vi "Errors Registered.vi"(8 "error in (no error)":errorcluster, 9 "Operation":T5, 11 "Error Info":T1 {"Context"."name" items=["Method Name", "Parameter Name", "VI Name", "Control Name", "Proxy Dll Path", "Project Library Name"]; "Error Number" items=["ERR_NOERROR"=0, "ERR_ACCESS_OUTPUTFOLDER"=1, "ERR_INVALID_LIBRARYNAME"=2, "ERR_CREATE_VIWRAPPER"=3, "ERR_UNKNOWN"=201, "ERR_BAD_ARGUMENT"=202, "ERR_URL_NOTFOUND_BADWSDL"=203, "ERR_BADLYFORMATTEDURL"=204, "ERR_BADHOSTNAME"=205, "ERR_BADDIRECTORY"=206, "ERR_UNAUTHORIZEDACCESS"=207, "ERR_CREATELIBRARY"=208, "ERR_COMPILEERROR"=209]}) -> (0 "error out":errorcluster, 3 "Array (out)":T1[](array[typedef]) {"Context"."name" items=["Method Name", "Parameter Name", "VI Name", "Control Name", "Proxy Dll Path", "Project Library Name"]; "Error Number" items=["ERR_NOERROR"=0, "ERR_ACCESS_OUTPUTFOLDER"=1, "ERR_INVALID_LIBRARYNAME"=2, "ERR_CREATE_VIWRAPPER"=3, "ERR_UNKNOWN"=201, "ERR_BAD_ARGUMENT"=202, "ERR_URL_NOTFOUND_BADWSDL"=203, "ERR_BADLYFORMATTEDURL"=204, "ERR_BADHOSTNAME"=205, "ERR_BADDIRECTORY"=206, "ERR_UNAUTHORIZEDACCESS"=207, "ERR_CREATELIBRARY"=208, "ERR_COMPILEERROR"=209]})   [LabVIEW 2020, in "WebServiceImporter.lvlib" / "Error Handling.lvlib"]
uses:
  <vilib>/Platform/WebService/Error Handling/Error Handling.lvlib
  <vilib>/Platform/WebService/Error Handling/Error/Operation.ctl
  <vilib>/Platform/WebService/Error Handling/Error/Error Info.ctl
  <vilib>/Platform/WebService/Error Handling/Error/Error Number.ctl
  <vilib>/Platform/WebService/Error Handling/Error/Context.ctl
  <vilib>/Platform/WebService/Error Handling/Error/Context Name.ctl
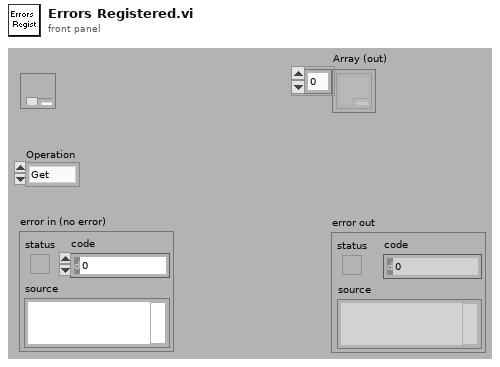
[diagram p1: front panel]
types:
  T1 = typedef "WebServiceImporter.lvlib/Error Handling.lvlib/Error Info.ctl" = cluster{"Specifics":string, "Error Number":T2, "Call Chain":string, "Context":T3}
  T2 = typedef "WebServiceImporter.lvlib/Error Handling.lvlib/Error Number.ctl" = u16
  T3 = typedef "WebServiceImporter.lvlib/Error Handling.lvlib/Context.ctl" = cluster{"name":T4, "value":string}[]
  T4 = typedef "WebServiceImporter.lvlib/Error Handling.lvlib/Context Name.ctl" = u16
  T5 = typedef "WebServiceImporter.lvlib/Error Handling.lvlib/Operation.ctl" = enum16{"Get", "Add", "Clear"}
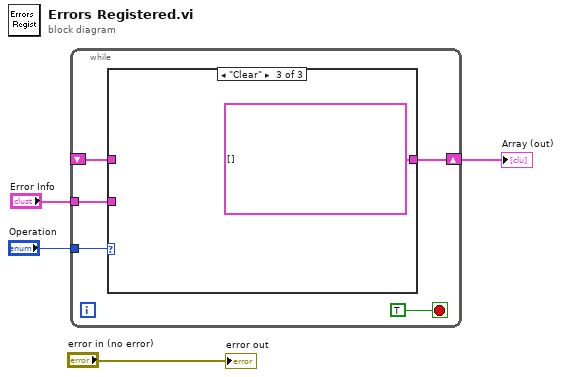
[diagram p0: block diagram]
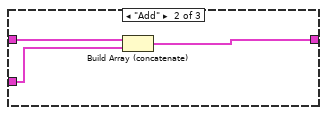
[diagram p3: hidden frame]
diagram:
  n1 = while {
    tunnel: "Operation" -> [w8]
    tunnel: "Error Info" -> [w7]
    shift-right: [w6] -> w1
    shift-left: _ -> [w5]
    stop <- TRUE stop-if-true
    n2 = case shown="\"Clear\"" w8 {
      tunnel: w7 -> [_ w13 _]
      tunnel: [w10 w12 T1[] []] -> w6
      tunnel: w5 -> [w10 w11 _]
      frame "Get", Default {
      }
      frame "Add" {
        n3 = Build Array (concatenate)(w11, w13) -> (w12:T1[])
      }
      frame "Clear" {
      }
    }
  }
  "Array (out)" <- w1
  "error out" <- "error in (no error)"
